vi "UDP_Server.vi"() -> ()   [LabVIEW 2020]
panel:
  in  "stop 2":bool
  out "data rx":string
  in  "data send":string
  in  "Puerto de Destino":u16
  in  "stop":bool
  # "Maquina 1"
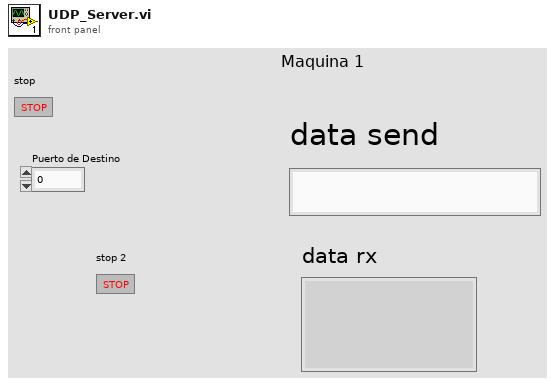
[diagram p1: front panel]
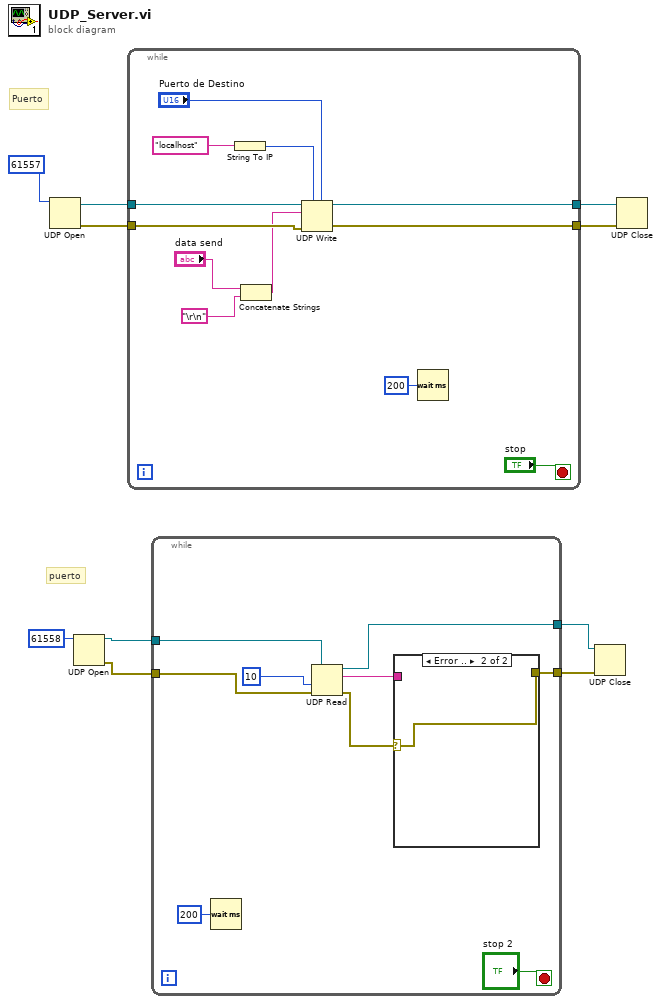
[diagram p0: block diagram]
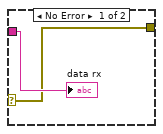
[diagram p2: hidden frame]
diagram:
  # "puerto"
  # "Puerto"
  n1 = UDP Open(11:u16 61557 ("port")) -> (port=w9:refnum<k16>, 0:w8:errorcluster)  [unwired: 4 in, 1 out]
  n2 = UDP Open(11:u16 61558 ("port")) -> (port=w5:refnum<k16>, 0:w4:errorcluster)  [unwired: 4 in, 1 out]
  n3 = while {
    tunnel: w9 -> [w21]
    tunnel: w8 -> [w20]
    tunnel: [w14] -> w7
    tunnel: [w13] -> w6
    stop <- "stop" stop-if-true
    n4 = String To IP(1:"localhost") -> (0:w19:u32)
    n5 = Concatenate Strings("data send", "\r\n") -> (w16:string)
    n6 = UDP Write(address=w19, port or service name="Puerto de Destino", connection ID=w21, data in=w16, 8:w20) -> (error out=w13:errorcluster, 3:w14:refnum<k16>)  [unwired: 1 in]
    n7 = Wait (ms)(milliseconds to wait=u32 200) -> ()  [unwired: 1 out]
  }
  n8 = while {
    tunnel: w5 -> [w30]
    tunnel: w4 -> [w29]
    tunnel: [w26] -> w3
    tunnel: [w24] -> w2
    stop <- "stop 2" stop-if-true
    n9 = Wait (ms)(milliseconds to wait=u32 200) -> ()  [unwired: 1 out]
    n10 = UDP Read(connection ID=w30, timeout ms (25000)=10, 8:w29) -> (data out=w25:string, error out=w27:errorcluster, 3:w26:refnum<k16>)  [unwired: 1 in, 2 out]
    n11 = case shown="Error .." w27 {
      selector: w27 -> [w32 w34]
      tunnel: w25 -> [w33 _]
      tunnel: [w32 w34] -> w24
      frame No Error {
        "data rx" <- w33
      }
      frame Error {
      }
    }
  }
  n12 = UDP Close(connection ID=w3, 8:w2) -> ()  [unwired: 2 out]
  n13 = UDP Close(connection ID=w7, 8:w6) -> ()  [unwired: 2 out]
